vi "setClockChans.vi"(0 "Analogue Data (volts)":dbl[][](array[numeric])) -> (1 "Modified Analogue Data (volts)":dbl[][](array[numeric]), 2 "MSB":dbl[](array[numeric]), 3 "LSB":dbl[](array[numeric]))   [LabVIEW 2013]
uses:
  Controls/chanType.ctl
  Globals/measurementGlobal.vi
panel:
  out "LSB":dbl[](graph)
  out "MSB":dbl[](graph)
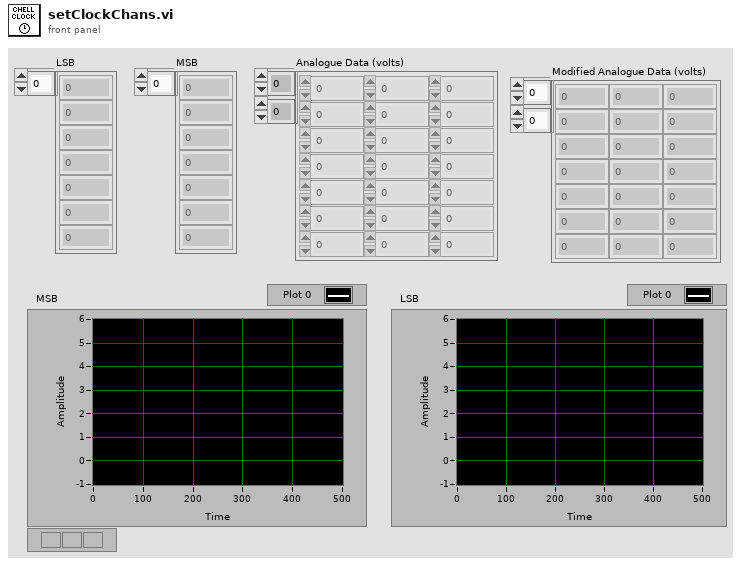
[diagram p1: front panel]
types:
  T1 = cluster{"Most Significant Bit":dbl, "Least Significant Bit":dbl}[]
  T2 = typedef "chanType.ctl" = enum16{"Default", "Clock", "Pressure Scanner"}
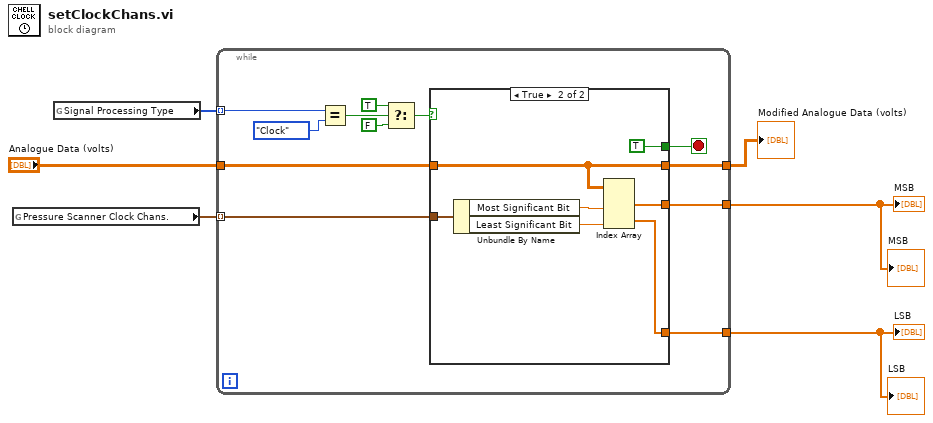
[diagram p0: block diagram]
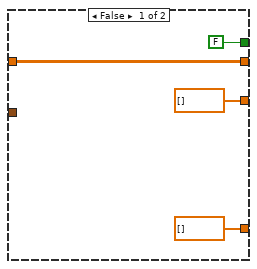
[diagram p2: hidden frame]
diagram:
  n1 = global read "measurementGlobal.vi" "Pressure Scanner Clock Chans."() -> (w6:T1)
  n2 = global read "measurementGlobal.vi" "Signal Processing Type"() -> (w2:T2[])
  n3 = while {
    tunnel: "Analogue Data (volts)" -> [w16]
    tunnel: w6 -> [w18] mode=indexing
    tunnel: [w14] -> w4
    tunnel: [w17] -> w3
    tunnel: [w15] -> w5
    tunnel: w2 -> [w8] mode=indexing
    stop <- w9 stop-if-true
    n4 = Equal?(x=w8, y=chanType."Clock") -> (x = y?=w13:bool)
    n5 = Select(t=TRUE, s=w13, f=FALSE) -> (s? t:f=w10:bool)
    n6 = case shown="True" w10 {
      tunnel: w18 -> [_ w29]
      tunnel: [dbl[] [] ("Analogue Data (volts)") w28] -> w17
      tunnel: w16 -> [w22 w23]
      tunnel: [w22 w23] -> w15
      tunnel: [dbl[] [] ("Analogue Data (volts)") w25] -> w14
      tunnel: [FALSE TRUE] -> w9
      frame False {
      }
      frame True {
        n7 = Unbundle By Name(w29) -> ("Most Significant Bit"=w27:dbl, "Least Significant Bit"=w26:dbl)
        n8 = Index Array(array=w23, index (col) #1=w27, index (col) #2=w26) -> (element #1=w25:dbl[], element #2=w28:dbl[])  [unwired: 2 in]
      }
    }
  }
  "MSB" <- w4
  "LSB" <- w3
  "Modified Analogue Data (volts)" <- w5
  "MSB" <- w4
  "LSB" <- w3
